vi "Configure Output Protection.vi"(6 "Compliance Voltage (2 V)":dbl=2.0, 7 "Enable Output Protection (T: Enable)":bool=TRUE, 8 "error in (no error)":errorcluster, 9 "Compliance Current (0.0001 A)":dbl=0.0001, 10 "Channel (0: Channel 1)":i32(ring) items=["Channel 1", "Channel 2"], 11 "VISA resource name":refnum<visa-resource-name>) -> (0 "error out":errorcluster, 3 "VISA resource name out":refnum<visa-resource-name>)   [LabVIEW 2023, in "Agilent B2900 Series.lvlib"]
doc: "Configures over current protection (OCP) and over voltage protection (OVP). Specify the output current limit value and the behavior of the power supply when the output current is greater than or equal to that value."
uses:
  Agilent B2900 Series.lvlib
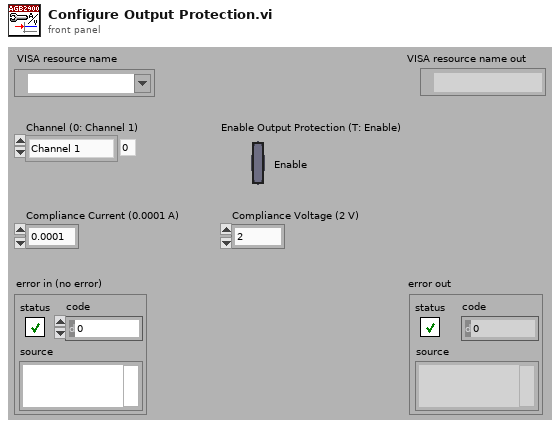
[diagram p1: front panel]
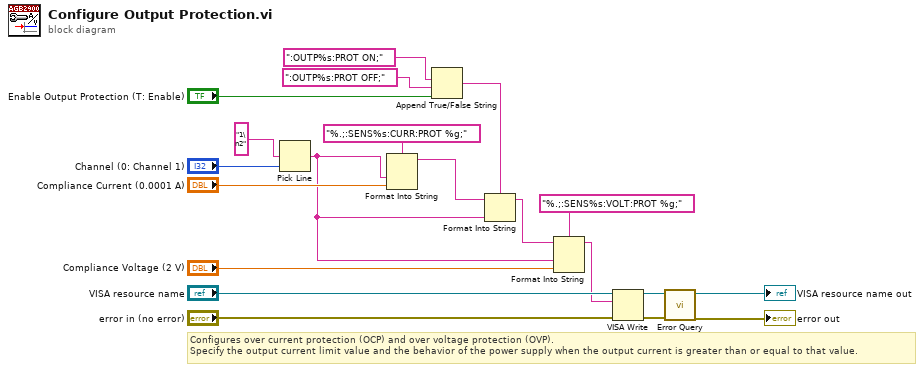
[diagram p0: block diagram]
diagram:
  # "Configures over current protection (OCP) and over voltage protection (OVP).  \nSpecify the output current limit value and the behavior of the power supply when the output current is greater than or equal to that value."
  n1 = Pick Line(multi-line string="1\n2" ("string (\"\")"), line index="Channel (0: Channel 1)") -> (output string=w1:string)  [unwired: 1 in]
  n2 = Format Into String(format string="%.;:SENS%s:CURR:PROT %g;", w1, "Compliance Current (0.0001 A)") -> (resulting string=w7:string)  [unwired: 2 in, 1 out]
  n3 = Append True/False String(1:"Enable Output Protection (T: Enable)", 2:":OUTP%s:PROT OFF;", 3:":OUTP%s:PROT ON;") -> (0:w6:string)  [unwired: 1 in]
  n4 = Format Into String(format string=w6, initial string=w7, w1) -> (resulting string=w2:string)  [unwired: 1 in, 1 out]
  n5 = Format Into String(format string="%.;:SENS%s:VOLT:PROT %g;", initial string=w2, w1, "Compliance Voltage (2 V)") -> (resulting string=w3:string)  [unwired: 1 in, 1 out]
  n6 = VISA Write(VISA resource name="VISA resource name", write buffer=w3, error in (no error)="error in (no error)") -> (VISA resource name out=w13:refnum<visa-resource-name>, error out=w12:errorcluster)  [unwired: 1 out]
  n7 = call "Error Query.vi"("error in (no error)"=w12, "VISA resource name"=w13) -> ("error out"=→"error out":errorcluster, "VISA resource name out"=→"VISA resource name out":refnum<visa-resource-name>)  [unwired: 6 in, 2 out]
